vi "Init.vi"(7 "MaxNumTimeouts (20)":u32=15, 8 "Error In":errorcluster, 11 "ChipKit Configuration":T1={"COM Port"="", "Board Type"=enum."ChipKit uC32", "Connection Type"=enum."USB / Serial", "Baud Rate (115200)"=115200, "Bytes Per Packet (15)"=15}) -> (0 "Error Out":errorcluster, 3 "ChipKit Configuration":T1={"COM Port"="", "Board Type"=enum."ChipKit Uno32", "Connection Type"=enum."USB / Serial", "Baud Rate (115200)"=115200, "Bytes Per Packet (15)"=15})   [LabVIEW 2011, in "LabVIEW Interface for ChipKit.lvlib"]
doc: "Initializes a connection to the Chipkit running the LabVIEW Interface for Chipkit firmware.\n\nNote: The baud rate specified must match the baud rate defined by DEFAULTBAUDRATE in the Chipkit firmware (115200 by default).\n\nNote: The Bytes Per Packet input must match the COMMANDLENGTH specified in the Arduino firmware (15 by default)."
uses:
  Private/Type Defs/Chipkit Resource.ctl
  Private/Type Defs/Board Type.ctl
  Private/Type Defs/Connection Type.ctl
  <vilib>/Instr/_visa.llb/VISA Configure Serial Port (Instr).vi
  LabVIEW Interface for ChipKit.lvlib
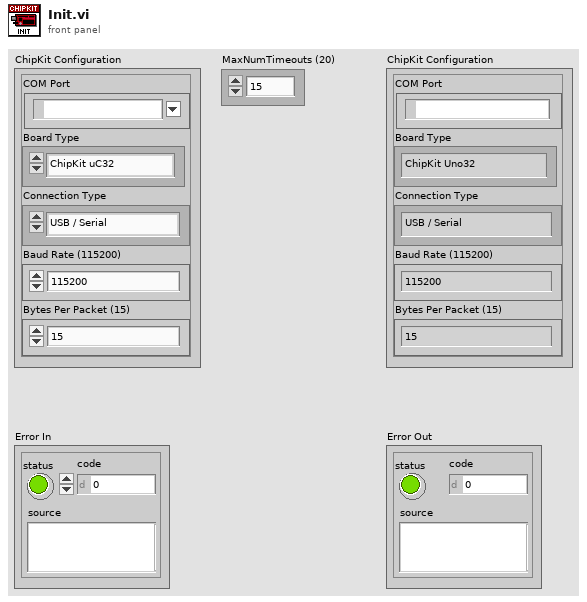
[diagram p1: front panel]
types:
  T1 = typedef "LabVIEW Interface for ChipKit.lvlib/Chipkit Resource.ctl" = cluster{"COM Port":refnum<visa-resource-name>, "Board Type":T2, "Connection Type":T3, "Baud Rate (115200)":u32, "Bytes Per Packet (15)":u32}
  T2 = typedef "LabVIEW Interface for ChipKit.lvlib/Board Type.ctl" = enum16{"ChipKit uC32", "ChipKit Uno32", "ChipKit Max32"}
  T3 = typedef "LabVIEW Interface for ChipKit.lvlib/Connection Type.ctl" = enum8{"USB / Serial", "XBEE", "BlueSmirf (Bluetooth)"}
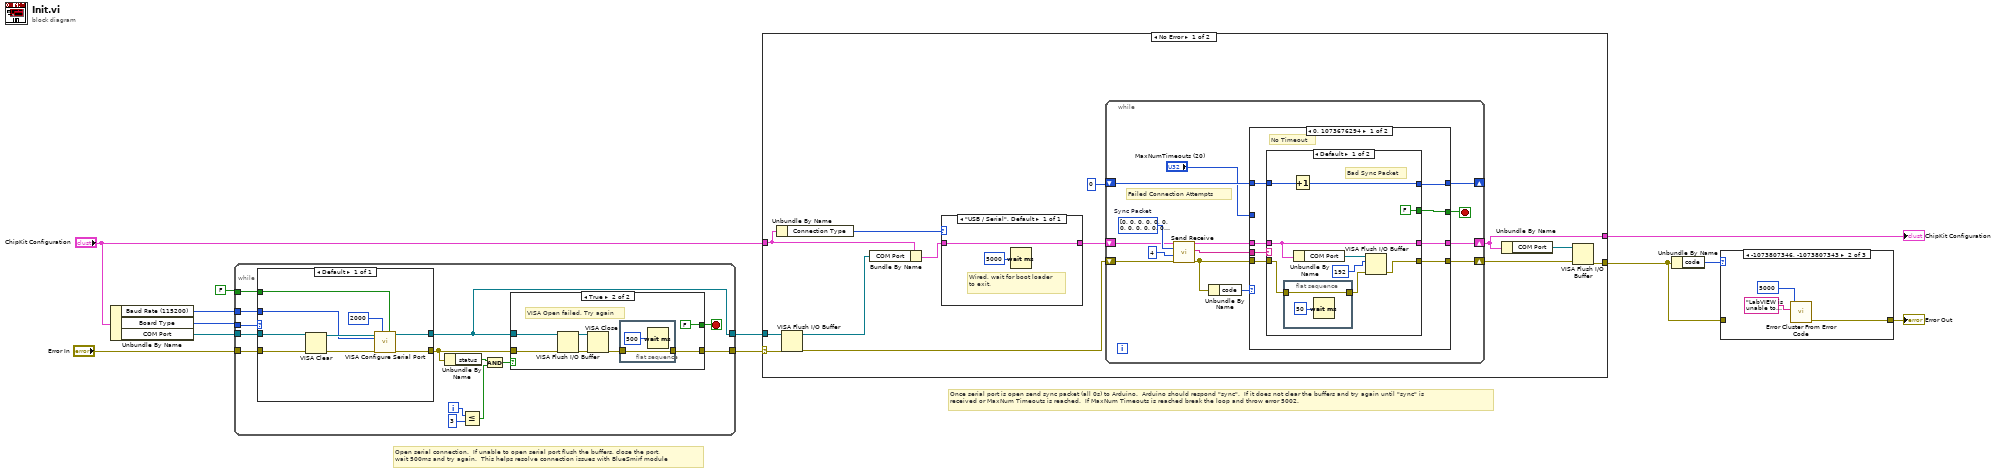
[diagram p0: block diagram]
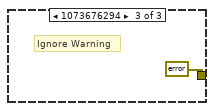
[diagram p3: hidden frame]
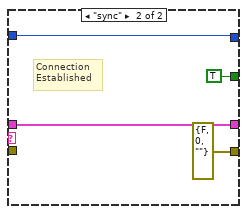
[diagram p4: hidden frame]
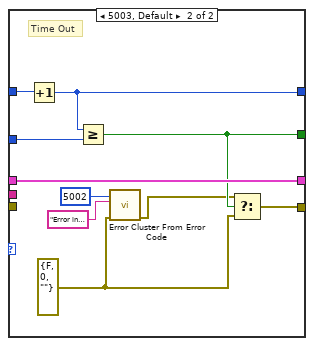
[diagram p5: hidden frame]
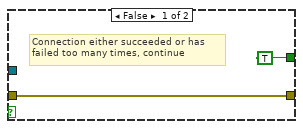
[diagram p7: hidden frame]
diagram:
  # "Once serial port is open send sync packet (all 0s) to Arduino.  Arduino should respond \"sync\".  If it does not clear the buffers and try again until \"sync\" is \nreceived or MaxNum Timeouts is reached.  If MaxNum Timeouts is reached break the loop and throw error 5002."
  # "Open serial connection.  If unable to open serial port flush the buffers, close the port,\nwait 500ms and try again.  This helps resolve connection issues with BlueSmirf module"
  n1 = Unbundle By Name("ChipKit Configuration") -> ("Baud Rate (115200)"=w4:u32, "Board Type"=w5:T2, "COM Port"=w7:refnum<visa-resource-name>)
  n2 = while {
    tunnel: FALSE ("Enable Termination\nChar (T)") -> [w26]
    tunnel: w7 -> [w15]
    tunnel: [w19] -> w11
    tunnel: [w17] -> w10
    tunnel: "Error In" -> [w16]
    tunnel: w5 -> [w14]
    tunnel: w4 -> [w13]
    i -> [w24]
    stop <- w18 stop-if-true
    n3 = case shown="Default" w14 {
      tunnel: w26 -> [w35]
      tunnel: [w34] -> w20
      tunnel: [w33] -> w17
      tunnel: w16 -> [w31]
      tunnel: w15 -> [w28]
      tunnel: w13 -> [w27]
      frame Default {
        n4 = VISA Clear(VISA resource name=w28, error in (no error)=w31) -> (VISA resource name out=w29:refnum<visa-resource-name>, error out=w30:errorcluster)
        n5 = call-poly "VISA Configure Serial Port"("VISA resource name"=w29, "timeout (10sec)"=u32 2000, "Enable Termination\nChar (T)"=w35, "baud rate (9600)"=w27, "error in (no error)"=w30) -> ("VISA resource name out"=w33:refnum<visa-resource-name>, "error out"=w34:errorcluster)  [unwired: 9 in]
      }
    }
    n6 = Unbundle By Name(w20) -> ("status"=w22:bool)
    n7 = Less Or Equal?(x=w24, y=3) -> (x <= y?=w23:bool)
    n8 = And(x=w22, y=w23) -> (x .and. y?=w21:bool)
    n9 = case shown="True" w21 {
      tunnel: w20 -> [w37 w40]
      tunnel: [w37 w39] -> w19
      tunnel: [TRUE FALSE] -> w18
      tunnel: w17 -> [_ w43]
      frame False {
        # "Connection either succeeded or has \nfailed too many times, continue"
      }
      frame True {
        # "VISA Open failed, Try again"
        n10 = VISA Flush I/O Buffer(VISA resource name=w43, error in (no error)=w40) -> (VISA resource name out=w42:refnum<visa-resource-name>, error out=w41:errorcluster)  [unwired: 1 in]
        n11 = VISA Close(VISA resource name=w42, error in (no error)=w41) -> (error out=w38:errorcluster)
        n12 = flat-sequence {
          tunnel: [w45] -> w39
          tunnel: w38 -> [w45]
          frame #0 {
            n13 = Wait (ms)(milliseconds to wait=u32 500) -> ()  [unwired: 1 out]
          }
        }
      }
    }
  }
  n14 = case shown="No Error" w11 {
    selector: w11 -> [w52 w110]
    tunnel: [w57 w109] -> w9
    tunnel: [w56 w110] -> w2
    tunnel: w10 -> [w54 _]
    tunnel: "ChipKit Configuration" -> [w48 w109]
    frame No Error {
      n15 = Unbundle By Name(w48) -> ("Connection Type"=w47:T3)
      n16 = VISA Flush I/O Buffer(VISA resource name=w54, error in (no error)=w52) -> (VISA resource name out=w49:refnum<visa-resource-name>, error out=w55:errorcluster)  [unwired: 1 in]
      n17 = Bundle By Name(cluster=w48, "COM Port"=w49) -> (w50:T1)
      n18 = case shown="\"USB / Serial\", Default" w47 {
        tunnel: w50 -> [w61]
        tunnel: [w61] -> w51
        frame "USB / Serial", Default {
          # "Wired, wait for boot loader\nto exit."
          n19 = Wait (ms)(milliseconds to wait=u32 5000) -> ()  [unwired: 1 out]
        }
      }
      n20 = while {
        shift-right: [w63] -> w57
        shift-left: w51 -> [w64]
        shift-right: [w68] -> w58
        shift-left: w55 -> [w75]
        shift-right: [w71] -> _
        shift-left: 0 -> [w70]
        stop <- w69 stop-if-true
        w74 = u8[] [0, 0, 0, 0, 0, 0, 0, 0, 0, 0, 0, 0, 0]  # Sync Packet
        # "Failed Connection Attempts"
        n21 = call "Send Receive.vi"("Error In"=w75, "Bytes To Read (0)"=u32 4, "Data"=w74, "ChipKit Resource"=w64) -> ("Error Out"=w65:errorcluster, "Read Buffer"=w66:string, "ChipKit Resource"=w67:T1)  [unwired: 5 in]
        n22 = Unbundle By Name(w65) -> ("code"=w72:i32)
        n23 = case shown="0, 1073676294" w72 {
          tunnel: [w79 w107] -> w71
          tunnel: w70 -> [w78 w108]
          tunnel: [w76 w105] -> w69
          tunnel: [w82 w103] -> w68
          tunnel: [w81 w106] -> w63
          tunnel: w67 -> [w80 w106]
          tunnel: w66 -> [w83 _]
          tunnel: w65 -> [w77 _]
          tunnel: "MaxNumTimeouts (20)" -> [_ w104]
          frame 0, 1073676294 {
            # "No Timeout"
            n24 = case shown="Default" w83 {
              tunnel: [w87 errorcluster {"status"=FALSE, "code"=0, "source"=""} ("error out")] -> w82
              tunnel: [w89 w97] -> w81
              tunnel: w80 -> [w89 w97]
              tunnel: [FALSE TRUE] -> w76
              tunnel: w78 -> [w91 w95]
              tunnel: [w90 w95] -> w79
              tunnel: w77 -> [w86 _]
              frame Default {
                # "Bad Sync Packet"
                n25 = flat-sequence {
                  tunnel: w86 -> [w93]
                  tunnel: [w93] -> w85
                  frame #0 {
                    n26 = Wait (ms)(milliseconds to wait=u32 50) -> ()  [unwired: 1 out]
                  }
                }
                n27 = Increment(x=w91) -> (x+1=w90:i32)
                n28 = Unbundle By Name(w89) -> ("COM Port"=w88:refnum<visa-resource-name>)
                n29 = VISA Flush I/O Buffer(VISA resource name=w88, mask (16)=u16 192, error in (no error)=w85) -> (error out=w87:errorcluster)  [unwired: 1 out]
              }
              frame "sync" {
                # "Connection \nEstablished"
              }
            }
          }
          frame 5003, Default {
            w99 = errorcluster {"status"=FALSE, "code"=0, "source"=""} ("f")
            # "Time Out"
            n30 = Increment(x=w108) -> (x+1=w107:i32)
            n31 = Greater Or Equal?(x=w107, y=w104) -> (x >= y?=w105:bool)
            n32 = call <vilib>:"Error Cluster From Error Code.vi"("error in (no error)"=w99, "error message (\"\")"="Error in Init.vi.  Unable to establish connection with ChipKit.  Please ensure that the correct COM port is specified and that the LabVIEW Interface for ChipKit firmware has been deployed to the ChipKit target." ("source"), "error code (0)"=5002) -> ("error out"=w100:errorcluster)  [unwired: 6 in]
            n33 = Select(t=w100, s=w105, f=w99) -> (s? t:f=w103:errorcluster)
          }
        }
      }
      n34 = Unbundle By Name(w57) -> ("COM Port"=w53:refnum<visa-resource-name>)
      n35 = VISA Flush I/O Buffer(VISA resource name=w53, error in (no error)=w58) -> (error out=w56:errorcluster)  [unwired: 1 in, 1 out]
    }
    frame Error {
    }
  }
  "ChipKit Configuration" <- w9
  n36 = Unbundle By Name(w2) -> ("code"=w3:i32)
  n37 = case shown="-1073807346, -1073807343" w3 {
    tunnel: w2 -> [w111 _ _]
    tunnel: [w111 w112 errorcluster {"status"=FALSE, "code"=0, "source"=""} ("error out")] -> w1
    frame 0, Default {
    }
    frame -1073807346, -1073807343 {
      n38 = call <vilib>:"Error Cluster From Error Code.vi"("error message (\"\")"="LabVIEW is unable to establish a connection with the ChipKit.  Please ensure that the correct COM Port, Board Type, and Baud Rate (default 115200) are specified in the Chipkit Configuration passed into the Init.vi." ("error message (\"\")"), "error code (0)"=5000) -> ("error out"=w112:errorcluster)  [unwired: 7 in]
    }
    frame 1073676294 {
      # "Ignore Warning"
    }
  }
  "Error Out" <- w1
